vi "Database.GetComponent.vi"(7 "Idx":i32, 8 "error in":errorcluster, 9 "Serial component":string, 10 "Ref component":string, 11 "Data in":T1) -> (0 "error out":errorcluster, 1 "Serial product":string, 2 "Ref product":string, 3 "Data out":T1)   [LabVIEW 2016]
uses:
  Database.Data.ctl
  Database.Data.Status.ctl
  Database.Data.Sets.ctl
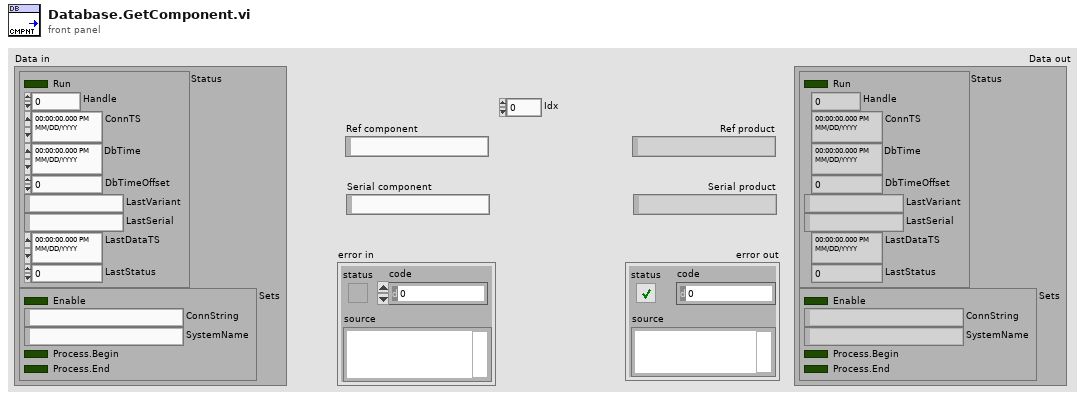
[diagram p1: front panel]
types:
  T1 = typedef "Database.Data.ctl" = cluster{"Status":T2, "Sets":T3}
  T2 = typedef "Database.Data.Status.ctl" = cluster{"Run":bool, "Handle":i32, "ConnTS":timestamp, "DbTime":timestamp, "DbTimeOffset":dbl, "LastVariant":string, "LastSerial":string, "LastDataTS":timestamp, "LastStatus":i32}
  T3 = typedef "Database.Data.Sets.ctl" = cluster{"Enable":bool, "ConnString":string, "SystemName":string, "Process.Begin":bool, "Process.End":bool}
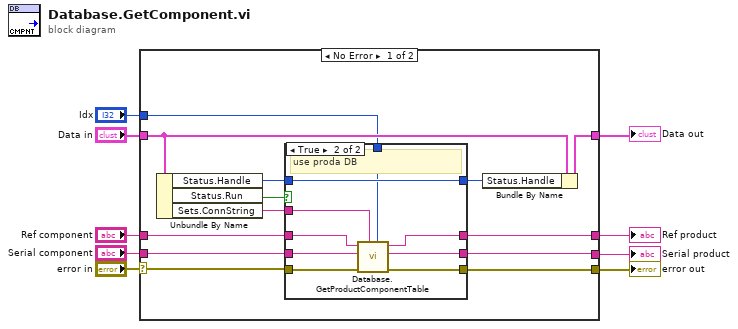
[diagram p0: block diagram]
diagram:
  n1 = case shown="No Error" "error in" {
    selector: "error in" -> [w22 w35]
    tunnel: [w13 w35] -> w9
    tunnel: "Data in" -> [w20 w34]
    tunnel: [w19 w34] -> w6
    tunnel: "Ref component" -> [w15 _]
    tunnel: "Serial component" -> [w14 _]
    tunnel: [w12 _] -> w3
    tunnel: [w11 _] -> w2
    tunnel: "Idx" -> [w10 _]
    frame No Error {
      n2 = Unbundle By Name(w20) -> ("Status.Handle"=w21:i32, "Status.Run"=w17:bool, "Sets.ConnString"=w16:string)
      n3 = case shown="True" w17 {
        tunnel: w22 -> [w24 w33]
        tunnel: w21 -> [w23 w29]
        tunnel: [w23 w29] -> w18
        tunnel: w16 -> [_ w32]
        tunnel: w15 -> [_ w31]
        tunnel: w14 -> [_ w30]
        tunnel: [w24 w28] -> w13
        tunnel: [_ w27] -> w12
        tunnel: [_ w26] -> w11
        tunnel: w10 -> [_ w25]
        frame False {
        }
        frame True {
          # "use proda DB"
          n4 = call "Database.GetProductComponentTable.vi"("Idx"=w25, "ConnectionString"=w32, "error in (no error)"=w33, "Component_SerialNo"=w30, "Component_WabcoNo"=w31) -> ("error out"=w28:errorcluster, "Product_SerialNo"=w27:string, "Product_WabcoNo"=w26:string)  [unwired: 3 in, 1 out]
        }
      }
      n5 = Bundle By Name(cluster=w20, "Status.Handle"=w18) -> (w19:T1)
    }
    frame Error {
    }
  }
  "error out" <- w9
  "Data out" <- w6
  "Ref product" <- w2
  "Serial product" <- w3
